vi "Pockels Cal-Power stepping sequence.vi"() -> (0 "Calibration points":i32=21 min=5 max=100, 1 "Pockels calibration voltage steps sequence (strings)":string[](array[string]), 2 "Voltage %":u16[](array[numeric]) format="%.0f%", 3 "Pockels calibration voltage steps sequence":dbl[](array[numeric]) format="%#_gV")   [LabVIEW 2013]
uses:
  Globals/gl_Calibration globals.vi
panel:
  out "size(s)":i32
  out "Increment":dbl format="%#_12f"
  # "Recommended numbers of calibration points are 11, 21, 41 etc such as the increment step is always a nice value rounded to two decimal points."
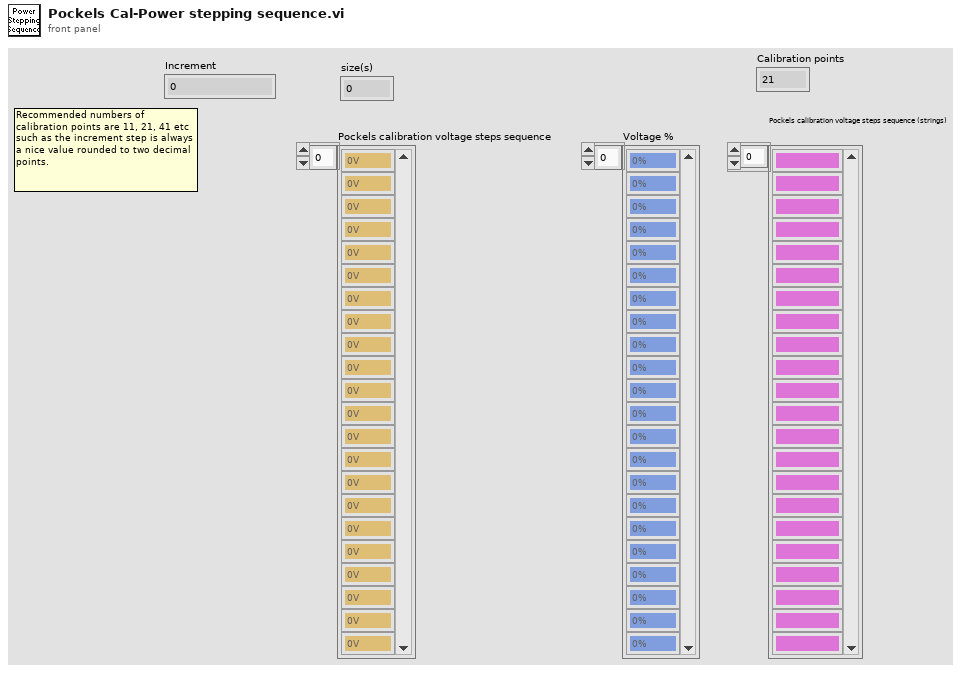
[diagram p1: front panel]
types:
  T1 = typedef "Cal points.ctl" = enum16{"5-points calibration (crude)", "11-points calibration", "21-points calibration", "41-points calibration"}
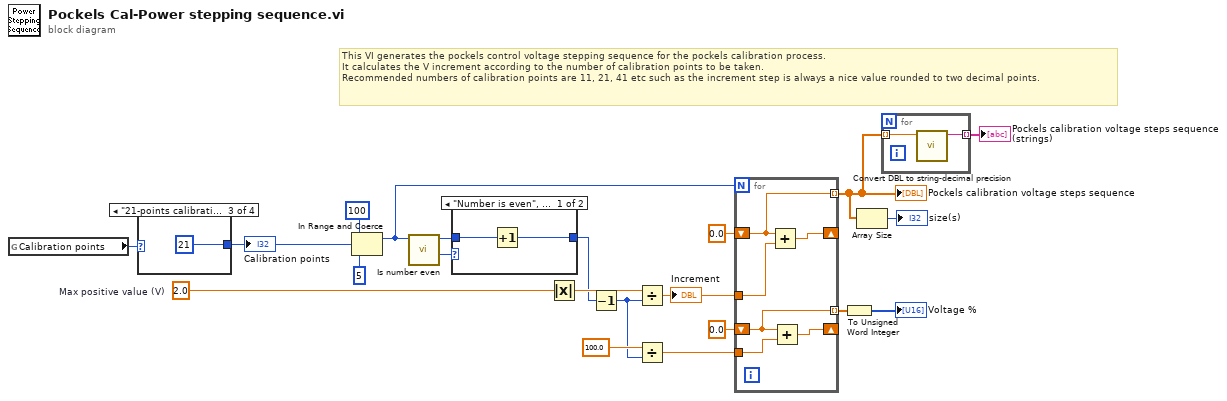
[diagram p0: block diagram]
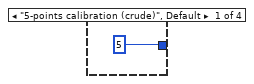
[diagram p2: hidden frame]
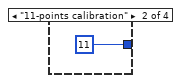
[diagram p3: hidden frame]
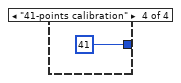
[diagram p4: hidden frame]
diagram:
  w1 = 2.0  # Max positive value (V)
  # "This VI generates the pockels control voltage stepping sequence for the pockels calibration process.\nIt calculates the V increment according to the number of calibration points to be taken.\nRecommended numbers of calibration points are 11, 21, 41 etc such as the increment step is always a nice value rounded to two decimal points."
  n1 = global read "gl_Calibration globals.vi" "Calibration points"() -> (w3:T1)
  n2 = case shown="\"21-points calibration\"" w3 {
    tunnel: [5 ("Calibration points") 11 ("Calibration points") 21 ("Calibration points") 41 ("Calibration points")] -> w2
    frame "5-points calibration (crude)", Default {
    }
    frame "11-points calibration" {
    }
    frame "21-points calibration" {
    }
    frame "41-points calibration" {
    }
  }
  "Calibration points" <- w2
  n3 = In Range and Coerce(upper limit=100, x=w2, lower limit=5) -> (coerced(x)=w14:i32)  [unwired: 1 out]
  n4 = call "Is number even.vi"("Number"=w14) -> ("Even/Odd"=w20:enum16{"Number is even", "Number is odd"}, "Number (dup)"=w15:i32)  [unwired: 9 in]
  n5 = case shown="\"Number is even\", Default" w20 {
    tunnel: [w26 w28] -> w16
    tunnel: w15 -> [w27 w28]
    frame "Number is even", Default {
      n6 = Increment(x=w27) -> (x+1=w26:i32)
    }
    frame "Number is odd" {
    }
  }
  n7 = Absolute Value(x=w1) -> (abs(x)=w19:dbl)
  n8 = Decrement(x=w16) -> (x-1=w8:i32)
  n9 = Divide(x=w19, y=w8) -> (x/y=w13:dbl)
  "Increment" <- w13
  n10 = Divide(x=100.0, y=w8) -> (x/y=w7:dbl)
  n11 = for {
    N: w14 -> [_]
    shift-right: [w33] -> _
    shift-left: 0.0 -> [w32]
    tunnel: w13 -> [w34]
    tunnel: [w32] -> w11 mode=indexing
    tunnel: w7 -> [w31]
    shift-right: [w30] -> _
    shift-left: 0.0 -> [w29]
    tunnel: [w29] -> w5 mode=indexing
    n12 = Add(x=w32, y=w34) -> (x+y=w33:dbl)
    n13 = Add(x=w29, y=w31) -> (x+y=w30:dbl)
  }
  "Pockels calibration voltage steps sequence" <- w11
  n14 = To Unsigned Word Integer(number=w5) -> (unsigned 16bit integer=→"Voltage %":u16[])
  n15 = Array Size(array=w11) -> (size(s)=→"size(s)":i32)
  n16 = for {
    tunnel: w11 -> [w36] mode=indexing
    tunnel: [w35] -> w10 mode=indexing
    n17 = call "Convert DBL to string-decimal precision.vi"("DBL Value"=w36) -> ("Converted to String"=w35:string)  [unwired: 10 in]
  }
  "Pockels calibration voltage steps sequence (strings)" <- w10
